vi "LabView360-5.vi"() -> ()   [LabVIEW 2017]
uses:
  <vilib>/Utility/file.llb/Write Delimited Spreadsheet (DBL).vi
panel:
  out "数组 2":dbl[][](array[numeric])
  in  "file path (dialog if empty) 2":path caption="文件路径 （空时为对话框）"
  in  "file path (dialog if empty)":path caption="文件路径 （空时为对话框）"
  out "数组":dbl[](array[numeric])
  out "Result":string caption="结果"
  out "子字符串":string
  out "连接的字符串":string
  out "长度":i32
  in  "字符串":string
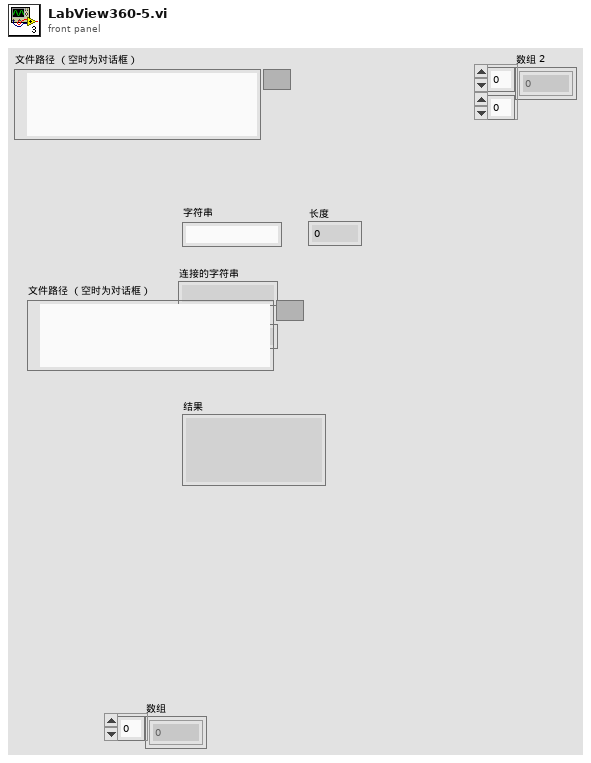
[diagram p1: front panel]
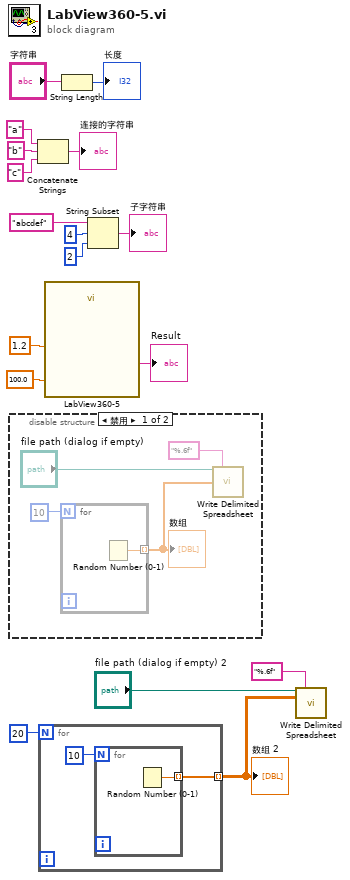
[diagram p0: block diagram]
diagram:
  n1 = disable-structure shown="禁用" {
    frame Disabled {
      n2 = for {
        N: 10 -> [_]
        tunnel: [w22] -> w20 mode=indexing
        n3 = Random Number (0-1)() -> (number: 0 to 1=w22:dbl)
      }
      "数组" <- w20
      n4 = call-poly <vilib>:"Write Delimited Spreadsheet.vi"("file path (dialog if empty)"="file path (dialog if empty)", "format (%.3f)"="%.6f", "1D data"=w20) -> ()  [unwired: 11 in, 2 out]
    }
    frame Enabled {
    }
  }
  n5 = Concatenate Strings("a", "b", "c") -> (→"连接的字符串":string)
  n6 = for {
    N: 20 -> [_]
    tunnel: [w23] -> w1 mode=indexing
    n7 = for {
      N: 10 -> [_]
      tunnel: [w25] -> w23 mode=indexing
      n8 = Random Number (0-1)() -> (number: 0 to 1=w25:dbl)
    }
  }
  "数组 2" <- w1
  n9 = call "LabView360-5.vi"("ch0"=1.2, "ch2"=100.0) -> ("Result"=→"Result":string)  [unwired: 12 in, 1 out]
  n10 = String Length(string="字符串") -> (length=→"长度":i32)
  n11 = String Subset(string="abcdef", offset (0)=4 ("偏移量(0)"), length (rest)=2 ("长度（剩余）")) -> (substring=→"子字符串":string)
  n12 = call-poly <vilib>:"Write Delimited Spreadsheet.vi"("file path (dialog if empty)"="file path (dialog if empty) 2", "format (%.3f)"="%.6f", "2D data"=w1) -> ()  [unwired: 11 in, 2 out]
